vi "get desired keys.vi"(8 "error in":errorcluster, 11 "Convert Bool to Velocity configuration in":refnum<class "Convert Bool to Velocity configuration.lvclass">) -> (0 "error out":errorcluster, 2 "desired keys":string[](array[string]), 3 "Convert Bool to Velocity configuration out":refnum<class "Convert Bool to Velocity configuration.lvclass">)   [LabVIEW 2017, in "Convert Bool to Velocity configuration.lvclass"]
uses:
  Convert Bool to Velocity configuration.lvclass
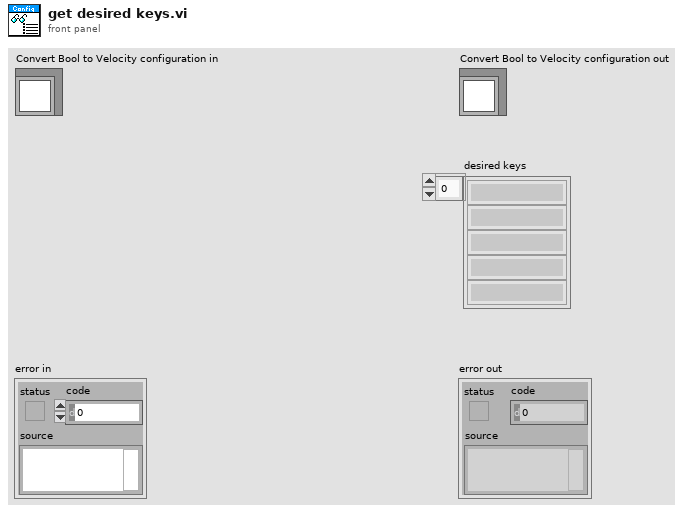
[diagram p1: front panel]
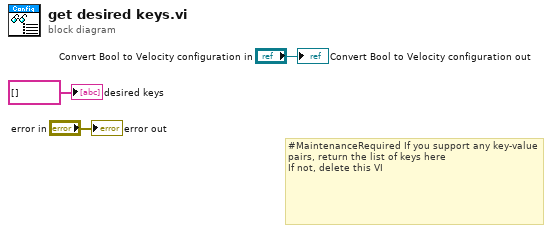
[diagram p0: block diagram]
diagram:
  # "#MaintenanceRequired If you support any key-value pairs, return the list of keys here\nIf not, delete this VI"
  "error out" <- "error in"
  "Convert Bool to Velocity configuration out" <- "Convert Bool to Velocity configuration in"
  "desired keys" <- string[] [] ("desired keys")
